vi "PH_Beamline.set States in GUI.vi"(0 "i ref in":refnum<vi>, 5 "error in":errorcluster) -> (14 "i ref out":refnum<vi>, 19 "error out":errorcluster)   [LabVIEW 2014, in "PH_Beamline.lvlib"]
uses:
  PH_Beamline.lvlib
  PH_BL-Master/PH_BL-Master.lvlib
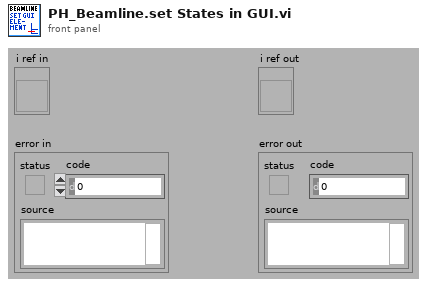
[diagram p1: front panel]
types:
  T1 = typedef "PH_BL-Master.lvlib/PH_BL-Master.i attribute.ctl" = cluster{"Remote controlled":bool, "Boolean Condition Service Subscriber":refnum<vi>[], "Picture Condition Service Subscriber":refnum<vi>[], "R2S":cluster{"GUI Ref":refnum<vi>, "State":bool}, "Vacua":cluster{"GUI Ref":refnum<vi>, "Limit":dbl, "Curr Value":dbl, "in range":bool}[], "O2 Inspection":cluster{"GUI Ref":refnum<vi>, "Concentration":dbl, "State":T2}[], "Boolean Status Service Subscriber":cluster{"GUI Ref":refnum<vi>, "Status":T2, "no Link?":bool, "Status Subscriber Class":T3}[], "Picture Status Service Subscriber":cluster{"GUI Ref":refnum<vi>, "Status":T2, "no Link?":bool, "Status Subscriber Class":T3}[], "6P 4Q Service Subscriber":cluster{"GUI Ref":refnum<vi>, "Selector":T4, "no Link?":bool}[], "Index of latest 6P 4Q changing Instance":i32, "Index of latest Picture Status changing Instance":i32, "Index of latest Boolean Status changing Instance":i32, "Vision ID on same Node":string, "Start Phase over?":bool, "GUI Ref Delete":refnum<vi>}
  T2 = typedef "PH_StatusHandler.lvlib/PH_StatusHandler.Status.ctl" = i16
  T3 = typedef "PH_BL-Master.lvlib/PH_BL-Master.Status Subscriber Class.ctl" = enum16{"unknown", "Switch", "BB", "6P Switch", "Switch GUI", "Switch and 6P State", "Force Sensor"}
  T4 = typedef "PH_4_Pos_Selector.lvlib/PH_4_Pos_Selector.Position Selector.ctl" = u16
  T5 = cluster{"GUI Ref":refnum<vi>, "Status":T2, "no Link?":bool, "Status Subscriber Class":T3}[]
  T6 = cluster{"GUI Ref":refnum<vi>, "Status":T2, "no Link?":bool, "Status Subscriber Class":T3}
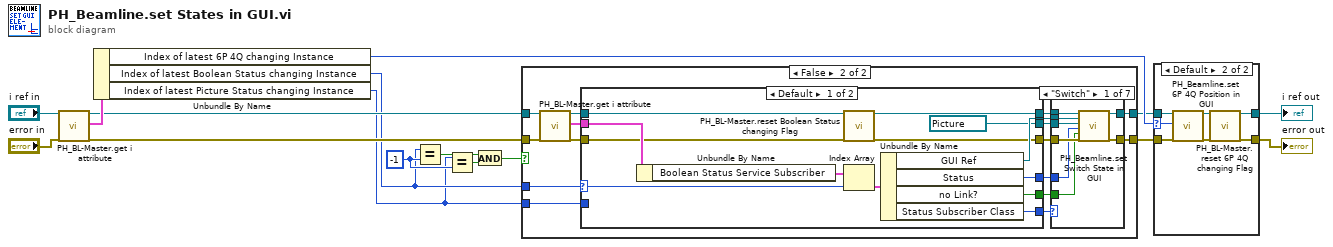
[diagram p0: block diagram]
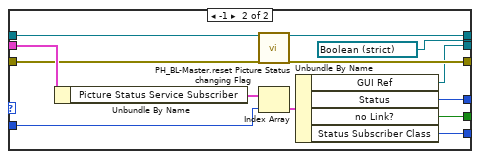
[diagram p3: hidden frame]
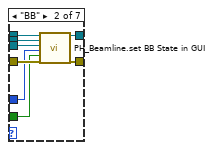
[diagram p4: hidden frame]
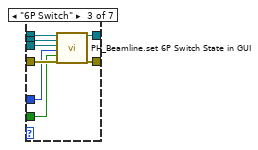
[diagram p5: hidden frame]
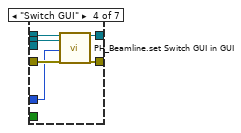
[diagram p6: hidden frame]
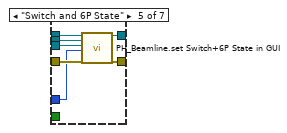
[diagram p7: hidden frame]
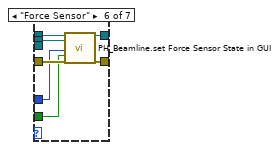
[diagram p8: hidden frame]
diagram:
  w10 = -1 ("y")
  n1 = call "PH_BL-Master.get i attribute.vi"("i ref in"="i ref in", "error in (no error)"="error in") -> ("i ref out"=w6:refnum<vi>, "i attribute"=w16:T1, "error out"=w7:errorcluster)  [unwired: 15 in]
  n2 = Unbundle By Name(w16) -> ("Index of latest 6P 4Q changing Instance"=w11:i32, "Index of latest Boolean Status changing Instance"=w3:i32, "Index of latest Picture Status changing Instance"=w2:i32)
  n3 = Equal?(x=w3, y=w10) -> (x = y?=w9:bool)
  n4 = Equal?(x=w2, y=w10) -> (x = y?=w8:bool)
  n5 = And(x=w9, y=w8) -> (x .and. y?=w1:bool)
  n6 = case shown="False" w1 {
    tunnel: [w18 w27] -> w5
    tunnel: [w17 w26] -> w4
    tunnel: w7 -> [w17 w34]
    tunnel: w6 -> [w18 w33]
    tunnel: w2 -> [_ w20]
    tunnel: w3 -> [_ w19]
    frame True {
    }
    frame False {
      n7 = call "PH_BL-Master.get i attribute.vi"("i ref in"=w33, "error in (no error)"=w34) -> ("i ref out"=w23:refnum<vi>, "i attribute"=w32:T1, "error out"=w25:errorcluster)  [unwired: 15 in]
      n8 = case shown="Default" w19 {
        selector: w19 -> [w35 _]
        tunnel: w32 -> [w47 w60]
        tunnel: [w44 w59] -> w31
        tunnel: [w43 w58] -> w30
        tunnel: [w42 w57] -> w29
        tunnel: [w41 refnum<vi> refnum ("GUI Ref")] -> w28
        tunnel: w25 -> [w40 w55]
        tunnel: [w39 w54] -> w24
        tunnel: w23 -> [w38 w53]
        tunnel: [w37 w52] -> w22
        tunnel: [refnum<vi> refnum ("Pic GUI Ref") w51] -> w21
        tunnel: w20 -> [_ w50]
        frame Default {
          n9 = Unbundle By Name(w47) -> ("Boolean Status Service Subscriber"=w46:T5)
          n10 = call "PH_BL-Master.reset Boolean Status changing Flag.vi"("i ref in"=w38, "error in"=w40) -> ("i ref out"=w37:refnum<vi>, "error out"=w39:errorcluster)  [unwired: 16 in]
          n11 = Index Array(array=w46, index=w35) -> (element=w45:T6)
          n12 = Unbundle By Name(w45) -> ("GUI Ref"=w41:refnum<vi>, "Status"=w42:T2, "no Link?"=w43:bool, "Status Subscriber Class"=w44:T3)
        }
        frame -1 {
          n13 = Unbundle By Name(w60) -> ("Picture Status Service Subscriber"=w49:T5)
          n14 = call "PH_BL-Master.reset Picture Status changing Flag.vi"("i ref in"=w53, "error in"=w55) -> ("i ref out"=w52:refnum<vi>, "error out"=w54:errorcluster)  [unwired: 16 in]
          n15 = Index Array(array=w49, index=w50) -> (element=w48:T6)
          n16 = Unbundle By Name(w48) -> ("GUI Ref"=w51:refnum<vi>, "Status"=w57:T2, "no Link?"=w58:bool, "Status Subscriber Class"=w59:T3)
        }
      }
      n17 = case shown="\"Switch\"" w31 {
        tunnel: [w67 w76 w84 w90 w97 w104 w106] -> w27
        tunnel: [w65 w75 w83 w89 w96 w103 w105] -> w26
        tunnel: w24 -> [w66 w74 w82 w88 w95 w102 w105]
        tunnel: w22 -> [w68 w73 w81 w87 w94 w101 w106]
        tunnel: w30 -> [w64 w69 w77 _ _ w98 _]
        tunnel: w29 -> [w63 w70 w78 w85 w91 w99 _]
        tunnel: w28 -> [w62 w72 w80 w86 w93 w100 _]
        tunnel: w21 -> [w61 w71 w79 _ w92 _ _]
        frame "Switch" {
          n18 = call "PH_Beamline.set Switch State in GUI.vi"("i ref in"=w68, "Boolean GUI Ref"=w62, "Picture GUI Ref"=w61, "Status"=w63, "no Link?"=w64, "error in (no error)"=w66) -> ("i ref out"=w67:refnum<vi>, "error out"=w65:errorcluster)  [unwired: 12 in]
        }
        frame "BB" {
          n19 = call "PH_Beamline.set BB State in GUI.vi"("i ref in"=w73, "Boolean GUI Ref"=w72, "Picture GUI Ref"=w71, "Status"=w70, "no Link?"=w69, "error in"=w74) -> ("i ref out"=w76:refnum<vi>, "error out"=w75:errorcluster)  [unwired: 12 in]
        }
        frame "6P Switch" {
          n20 = call "PH_Beamline.set 6P Switch State in GUI.vi"("i ref in"=w81, "Boolean GUI Ref"=w80, "Picture GUI Ref"=w79, "Status"=w78, "no Link?"=w77, "error in"=w82) -> ("i ref out"=w84:refnum<vi>, "error out"=w83:errorcluster)  [unwired: 12 in]
        }
        frame "Switch GUI" {
          n21 = call "PH_Beamline.set Switch GUI in GUI.vi"("i ref in"=w87, "Boolean GUI Ref"=w86, "Status"=w85, "error in"=w88) -> ("i ref out"=w90:refnum<vi>, "error out"=w89:errorcluster)  [unwired: 14 in]
        }
        frame "Switch and 6P State" {
          n22 = call "PH_Beamline.set Switch+6P State in GUI.vi"("i ref in"=w94, "Boolean GUI Ref"=w93, "Picture GUI Ref"=w92, "Subscriber State"=w91, "error in (no error)"=w95) -> ("i ref out"=w97:refnum<vi>, "error out"=w96:errorcluster)  [unwired: 13 in]
        }
        frame "Force Sensor" {
          n23 = call "PH_Beamline.set Force Sensor State in GUI.vi"("i ref in"=w101, "Force Sensor GUI Ref"=w100, "Subscriber State"=w99, "No Link"=w98, "error in (no error)"=w102) -> ("i ref out"=w104:refnum<vi>, "error out"=w103:errorcluster)  [unwired: 13 in]
        }
        frame Default {
        }
      }
    }
  }
  n24 = case shown="Default" w11 {
    selector: w11 -> [_ w110]
    tunnel: w4 -> [w107 w115]
    tunnel: [w107 w114] -> w13
    tunnel: w5 -> [w108 w112]
    tunnel: [w108 w113] -> w12
    frame -1 {
    }
    frame Default {
      n25 = call "PH_Beamline.set 6P 4Q Position in GUI.vi"("VI in"=w112, "Index 6P 4Q Instance to change"=w110, "error in (no error)"=w115) -> ("VI out"=w111:refnum<vi>, "error out"=w109:errorcluster)  [unwired: 15 in]
      n26 = call "PH_BL-Master.reset 6P 4Q changing Flag.vi"("i ref in"=w111, "error in"=w109) -> ("i ref out"=w113:refnum<vi>, "error out"=w114:errorcluster)  [unwired: 16 in]
    }
  }
  "error out" <- w13
  "i ref out" <- w12
